vi "Color Hex Code To Color Box.vi"(11 "Color Hex Code":string) -> (3 "Color":u32(colorbox))   [LabVIEW 2021]
panel:
  out "Active Cell:Cell Background Color":u32(colorbox)
  out "Numeric":u32
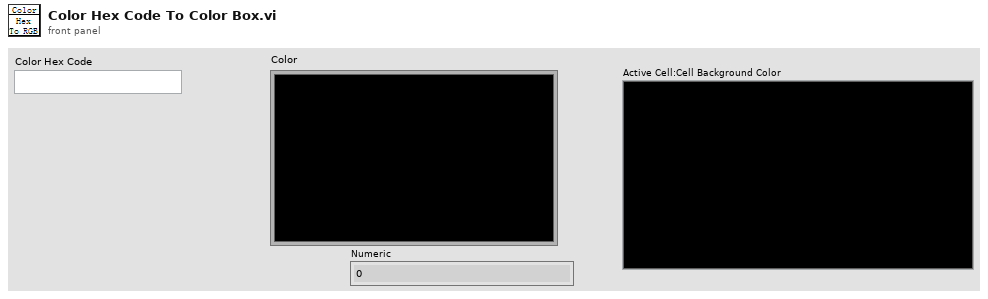
[diagram p1: front panel]
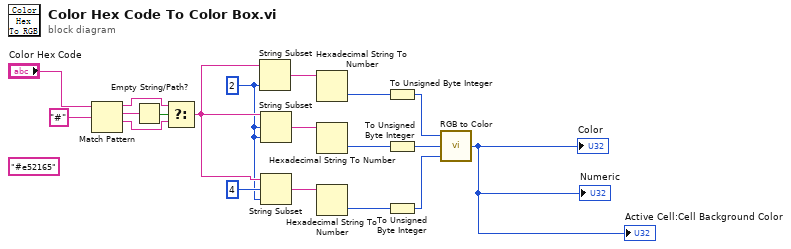
[diagram p0: block diagram]
diagram:
  w3 = 2 ("length (rest)")
  (unwired) "#e52165" ("node ID")
  n1 = Match Pattern(string="Color Hex Code", regular expression="#") -> (before substring=w17:string, match substring=w15:string, after substring=w18:string)  [unwired: 1 in, 1 out]
  n2 = Empty String/Path?(string/path=w15) -> (empty?=w16:bool)
  n3 = Select(t=w17, s=w16, f=w18) -> (s? t:f=w19:string)
  n4 = String Subset(string=w19, length (rest)=w3) -> (substring=w5:string)  [unwired: 1 in]
  n5 = String Subset(string=w19, offset (0)=w3, length (rest)=w3) -> (substring=w6:string)
  n6 = String Subset(string=w19, offset (0)=4, length (rest)=w3) -> (substring=w7:string)
  n7 = Hexadecimal String To Number(string=w5) -> (number=w8:u32)  [unwired: 2 in, 1 out]
  n8 = Hexadecimal String To Number(string=w6) -> (number=w9:u32)  [unwired: 2 in, 1 out]
  n9 = Hexadecimal String To Number(string=w7) -> (number=w12:u32)  [unwired: 2 in, 1 out]
  n10 = To Unsigned Byte Integer(number=w8) -> (unsigned 8bit integer=w10:u8)
  n11 = To Unsigned Byte Integer(number=w9) -> (unsigned 8bit integer=w11:u8)
  n12 = To Unsigned Byte Integer(number=w12) -> (unsigned 8bit integer=w13:u8)
  n13 = call <vilib>:"RGB to Color.vi"("B"=w13, "G"=w11, "R"=w10) -> ("Color"=→"Color" →"Numeric" →"Active Cell:Cell Background Color":u32)
